vi "generate_spatial_calibration_pattern.vi"(6 "Color Pixel Value":u32(colorbox)=65280, 8 "error in (no error)":errorcluster, 9 "Dot Radius (Projector Pixels)":i32, 10 "Points Array":cluster{"X":dbl, "Y":dbl}[](array[cluster]), 11 "StimulusImageIn":T1) -> (0 "error out":errorcluster, 3 "StimulusImageOut":T1)   [LabVIEW 2019]
uses:
  <vilib>/vision/Image Controls.llb/IMAQ Image.ctl
  <vilib>/vision/NI_Vision_Development_Module.lvlib
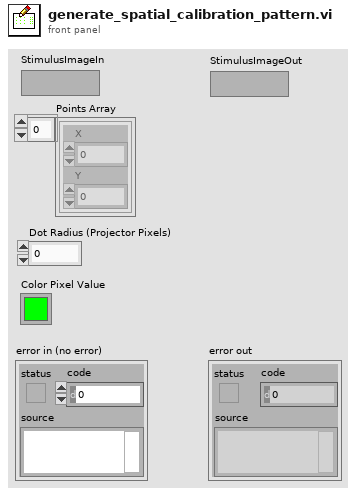
[diagram p1: front panel]
types:
  T1 = typedef "IMAQ Image.ctl" = refnum<image>
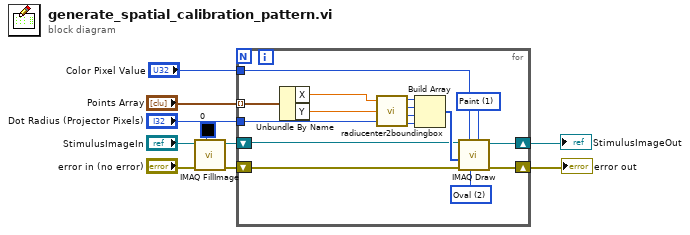
[diagram p0: block diagram]
diagram:
  n1 = call "IMAQ FillImage"("Color Pixel Value"=u32 0, "error in (no error)"="error in (no error)", "Image"="StimulusImageIn") -> ("error out"=w4:errorcluster, "Image Out"=w5:T1)  [unwired: 7 in]
  n2 = for {
    shift-right: [w18] -> w8
    shift-left: w5 -> [w19]
    shift-right: [w17] -> w9
    shift-left: w4 -> [w13]
    tunnel: "Dot Radius (Projector Pixels)" -> [w16]
    tunnel: "Points Array" -> [w12] mode=indexing
    tunnel: "Color Pixel Value" -> [w11]
    w26 = u16 1 items=["Frame", "Paint", "Invert Frame", "Invert Paint"] ("Draw Mode")
    w25 = u16 2 items=["Line", "Rectangle", "Oval"] ("Shape to draw")
    n3 = Unbundle By Name(w12) -> ("X"=w15:dbl, "Y"=w14:dbl)
    n4 = call "radiucenter2boundingbox.vi"("Radius"=w16, "ycenter"=w14, "xcenter"=w15) -> ("Bottom"=w20:i32, "Right"=w21:i32, "Top"=w22:i32, "Left"=w23:i32)  [unwired: 2 in]
    n5 = Build Array(w23, w22, w21, w20) -> (w24:i32[])
    n6 = call "IMAQ Draw"("Draw Mode"=w26, "Shape to draw"=w25, "Pixel Color"=w11, "error in (no error)"=w13, "Coordinates"=w24, "Image Src"=w19) -> ("error out"=w17:errorcluster, "Image Dst Out"=w18:T1)  [unwired: 4 in]
  }
  "StimulusImageOut" <- w8
  "error out" <- w9
